vi "Add-tab-cluster-controls.vi"(8 "error in (no error)":errorcluster, 11 "Controls in":refnum<vi>[](array[refnum])) -> (0 "error out":errorcluster, 3 "Controls out":refnum<vi>[](array[refnum]))   [LabVIEW 2013, in "SLMControl.lvlib" / "SC-UI.lvclass"]
uses:
  SC-UI.lvclass
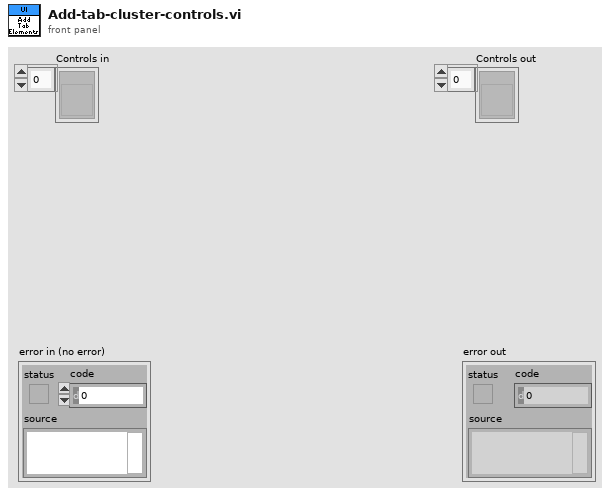
[diagram p1: front panel]
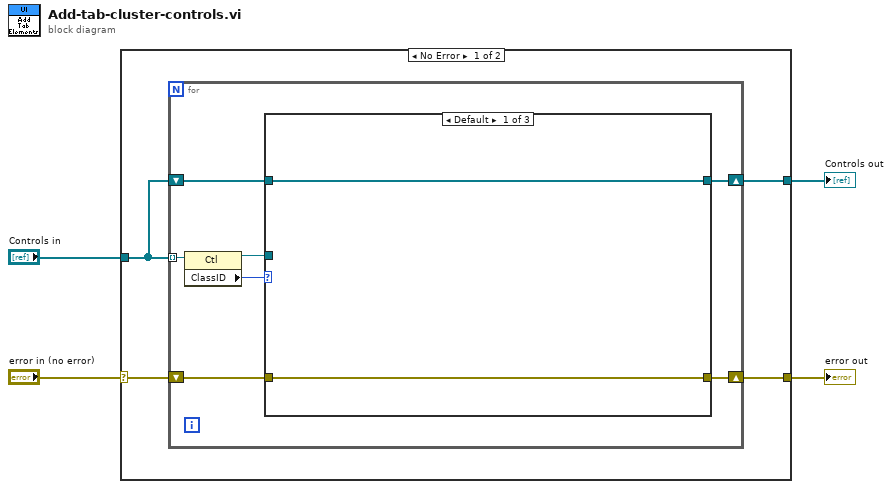
[diagram p0: block diagram]
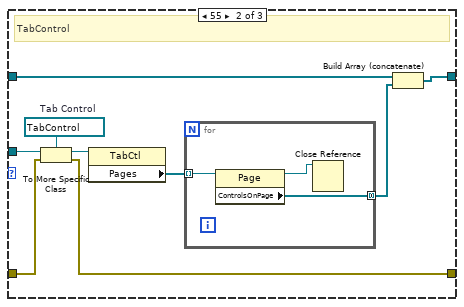
[diagram p2: hidden frame]
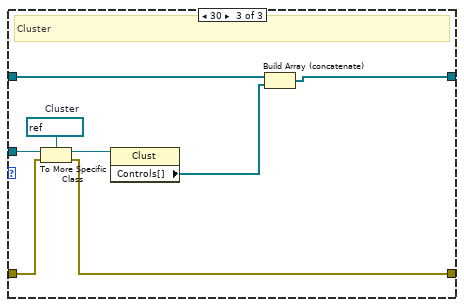
[diagram p3: hidden frame]
diagram:
  n1 = case shown="No Error" "error in (no error)" {
    selector: "error in (no error)" -> [w8 w39]
    tunnel: [w6 w39] -> w3
    tunnel: "Controls in" -> [w5 w38]
    tunnel: [w7 w38] -> w1
    frame No Error {
      n2 = for {
        tunnel: w5 -> [w15] mode=indexing
        shift-right: [w11] -> w7
        shift-left: w5 -> [w12]
        shift-right: [w9] -> w6
        shift-left: w8 -> [w10]
        n3 = property class="Ctl"(reference=w15) -> (reference out=w14:refnum<vi>, "ClassID"=w13:u32)  [unwired: 1 in, 1 out]
        n4 = case shown="Default" w13 {
          tunnel: w14 -> [_ w20 w34]
          tunnel: w12 -> [w17 w23 w36]
          tunnel: [w17 w22 w35] -> w11
          tunnel: w10 -> [w16 w19 w31]
          tunnel: [w16 w18 w30] -> w9
          frame Default {
          }
          frame 55 {
            w26 = refnum<vi> refnum  # Tab Control
            # "TabControl"
            n5 = To More Specific Class(target class=w26, reference=w20, error in=w19) -> (specific class reference=w25:refnum<vi>, error out=w18:errorcluster)
            n6 = property class="TabCtl"(reference=w25) -> ("Pages"=w24:refnum<vi>[])  [unwired: 1 in, 2 out]
            n7 = for {
              tunnel: w24 -> [w29] mode=indexing
              tunnel: [w28] -> w21 mode=concatenating
              n8 = property class="Page"(reference=w29) -> (reference out=w27:refnum<vi>, "ControlsOnPage"=w28:refnum<vi>[])  [unwired: 1 in, 1 out]
              n9 = Close Reference(reference=w27) -> ()  [unwired: 1 in, 1 out]
            }
            n10 = Build Array (concatenate)(w23, w21) -> (w22:refnum<vi>[])
          }
          frame 30 {
            w33 = refnum<vi> refnum  # Cluster
            # "Cluster"
            n11 = To More Specific Class(target class=w33, reference=w34, error in=w31) -> (specific class reference=w37:refnum<vi>, error out=w30:errorcluster)
            n12 = property class="Clust"(reference=w37) -> ("Controls[]"=w32:refnum<vi>[])  [unwired: 1 in, 2 out]
            n13 = Build Array (concatenate)(w36, w32) -> (w35:refnum<vi>[])
          }
        }
      }
    }
    frame Error {
    }
  }
  "error out" <- w3
  "Controls out" <- w1
